vi "Exemple_Preprocessing_OrdinalEncoder.vi"() -> ()   [LabVIEW 2020]
uses:
  Objet/6 - Datasets Transformation/6.3 - Processing Data/OrdinalEncoder/OrdinalEncoder.lvclass
panel:
  in  "y":string[][](array[string])
  in  "X":string[][](array[string])=[["Male", "1"], ["Female", "3"], ["Female", "2"]]
  out "Data":T1
  out "error out":errorcluster
  in  "error in":errorcluster caption="entrée d'erreur"
  in  "OrdinalEncoder":cluster{"dtype":string}={"dtype"="float"}
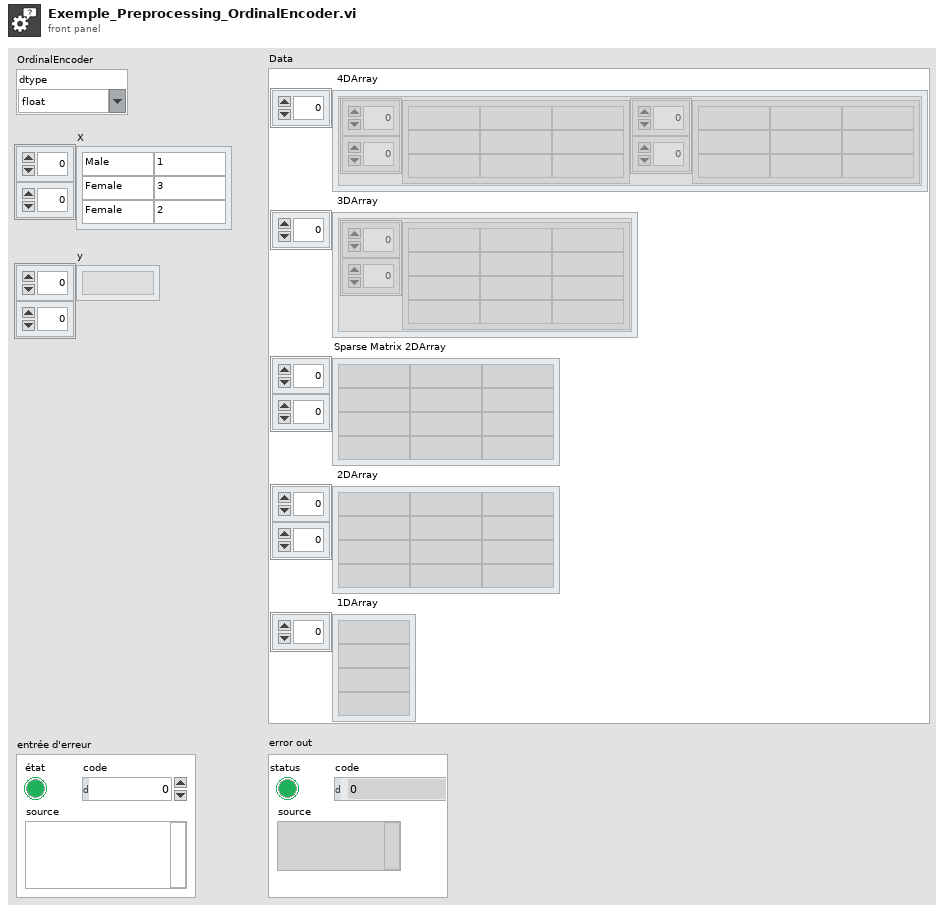
[diagram p1: front panel]
types:
  T1 = cluster{" 4DArray":cluster{"1":string[][], "2":string[][]}[], " 3DArray":cluster{"Tableau":string[][]}[], "Sparse Matrix 2DArray":string[][], " 2DArray":string[][], " 1DArray":string[]}
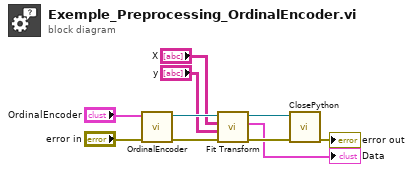
[diagram p0: block diagram]
diagram:
  n1 = call "OrdinalEncoder.vi"("error in (no error)"="error in", "OrdinalEncoder"="OrdinalEncoder") -> ("error out"=w8:errorcluster, "OrdinalEncoder.lvclass"=w7:refnum<class "OrdinalEncoder.lvclass">)  [unwired: 8 in]
  n2 = call-dynamic "Fit Transform.vi"("error in (no error)"=w8, "y"="y", "X"="X", "OrdinalEncoder.lvclass"=w7) -> ("error out"=w4:errorcluster, "Data"=→"Data":T1, "OrdinalEncoder.lvclass"=w3:refnum<class "OrdinalEncoder.lvclass">)  [unwired: 5 in]
  n3 = call-dynamic "ClosePython.vi"("error in (no error)"=w4, "Scikit-learn en entrée"=w3) -> ("error out"=→"error out":errorcluster)  [unwired: 8 in, 1 out]
